vi "sortSTData.vi"(8 "error in (no error)":errorcluster, 9 "channelData":T1(array[cluster]), 10 "times":dbl[](array[numeric]), 11 "ScriptEventList in":refnum<class "ScriptEventList.lvclass">) -> (0 "error out":errorcluster, 2 "sortedData":T1(array[cluster]), 3 "ScriptEventList out":refnum<class "ScriptEventList.lvclass">)   [LabVIEW 2011, in "Tools.lvlib" / "Scripting.lvlib" / "ScriptEventList.lvclass"]
uses:
  ScriptEventList.lvclass
  DatabaseHelpers/Database Objects/Channel/Channel.lvclass
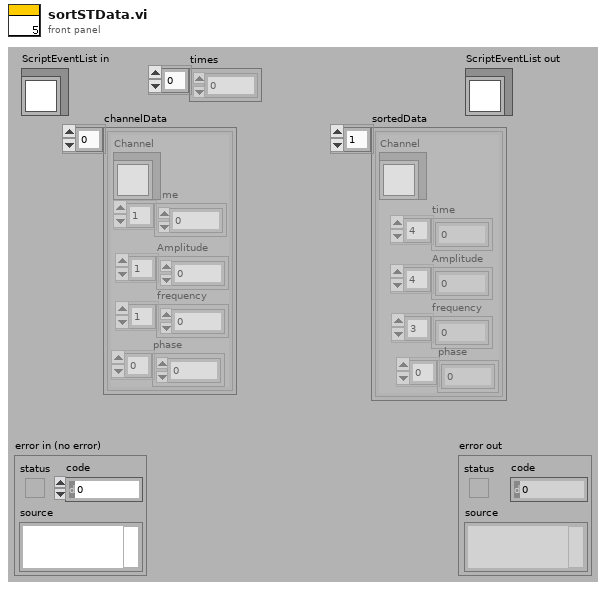
[diagram p1: front panel]
types:
  T1 = cluster{"Channel":refnum<class "Channel.lvclass">, "time":dbl[], "Amplitude":dbl[], "frequency":dbl[], "phase":dbl[]}[]
  T2 = cluster{"Channel":refnum<class "Channel.lvclass">, "time":dbl[], "Amplitude":dbl[], "frequency":dbl[], "phase":dbl[]}
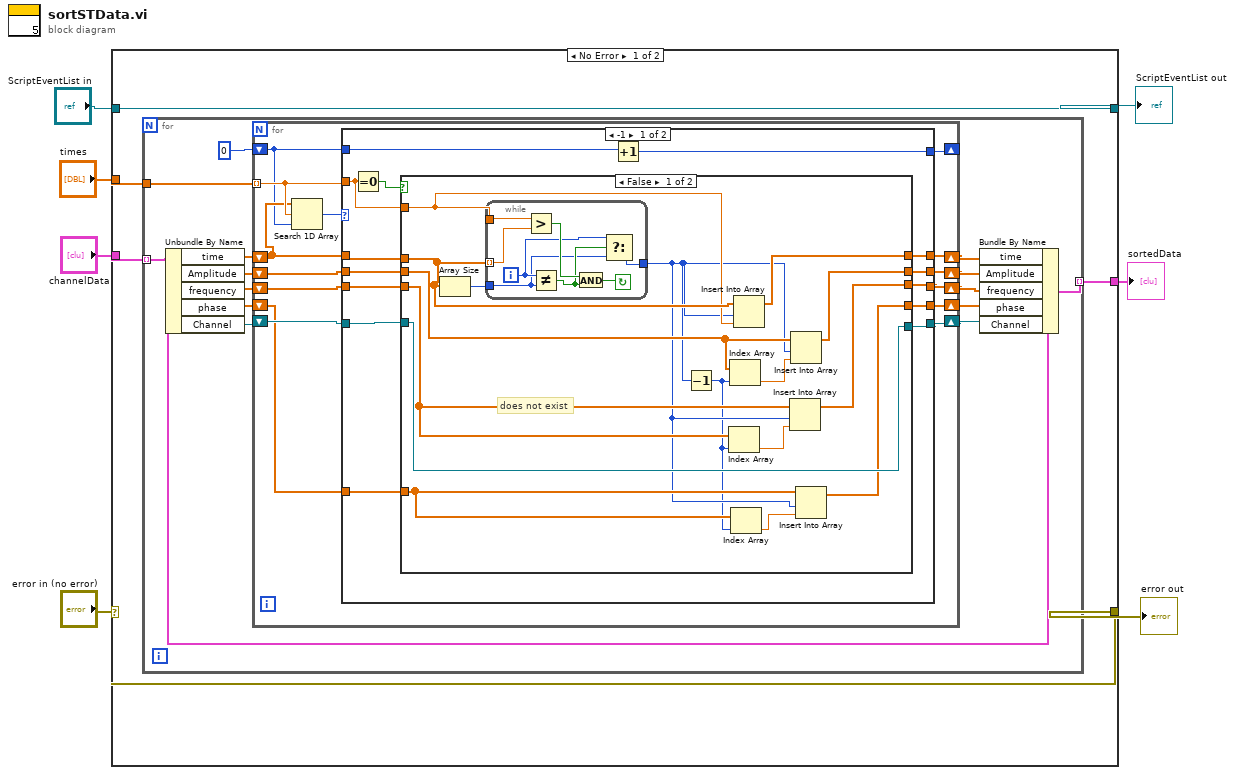
[diagram p0: block diagram]
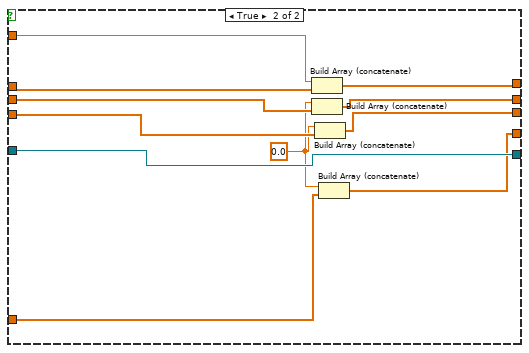
[diagram p2: hidden frame]
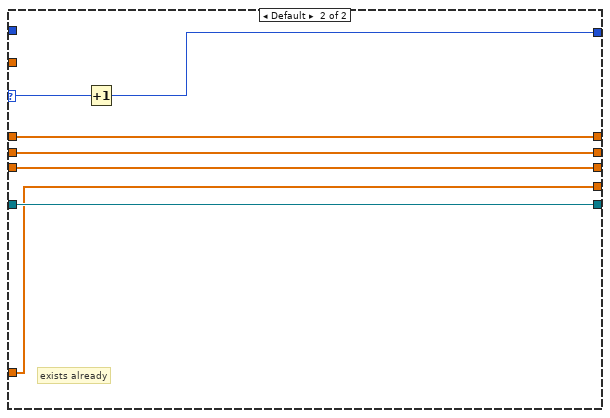
[diagram p3: hidden frame]
diagram:
  n1 = case shown="No Error" "error in (no error)" {
    selector: "error in (no error)" -> [w11 w98]
    tunnel: [w11 w98] -> w6
    tunnel: [w12 w97] -> w4
    tunnel: "ScriptEventList in" -> [w12 w97]
    tunnel: "times" -> [w9 _]
    tunnel: "channelData" -> [w10 _]
    tunnel: [w8 _] -> w1
    frame No Error {
      n2 = for {
        tunnel: w10 -> [w21] mode=indexing
        tunnel: w9 -> [w26]
        tunnel: [w17] -> w8 mode=indexing
        n3 = Unbundle By Name(w21) -> ("time"=w23:dbl[], "Amplitude"=w25:dbl[], "frequency"=w24:dbl[], "phase"=w15:dbl[], "Channel"=w16:refnum<class "Channel.lvclass">)
        n4 = for {
          tunnel: w26 -> [w32] mode=indexing
          shift-right: [w33] -> w20
          shift-left: w23 -> [w31]
          shift-right: [w34] -> w19
          shift-left: w25 -> [w39]
          shift-right: [w35] -> w18
          shift-left: w24 -> [w38]
          shift-right: [w36] -> w14
          shift-left: w16 -> [w37]
          shift-right: [w29] -> _
          shift-left: 0 -> [w30]
          shift-right: [w27] -> w13
          shift-left: w15 -> [w28]
          n5 = Search 1D Array(1D array=w31, element=w32, start index (0)=w30) -> (index of element=w40:i32)
          n6 = case shown="-1" w40 {
            selector: w40 -> [_ w92]
            tunnel: w31 -> [w52 w93]
            tunnel: w39 -> [w51 w94]
            tunnel: w38 -> [w50 w95]
            tunnel: w37 -> [w49 w96]
            tunnel: [w45 w96] -> w36
            tunnel: [w46 w95] -> w35
            tunnel: [w47 w94] -> w34
            tunnel: [w48 w93] -> w33
            tunnel: w32 -> [w53 _]
            tunnel: w30 -> [w44 _]
            tunnel: [w43 w91] -> w29
            tunnel: w28 -> [w42 w90]
            tunnel: [w41 w90] -> w27
            frame -1 {
              # "does not exist"
              n7 = Equal To 0?(x=w53) -> (x = 0?=w54:bool)
              n8 = case shown="False" w54 {
                tunnel: w53 -> [w69 w87]
                tunnel: w52 -> [w70 w89]
                tunnel: w51 -> [w67 w86]
                tunnel: w50 -> [w63 w84]
                tunnel: w49 -> [w61 w82]
                tunnel: [w68 w88] -> w48
                tunnel: [w65 w85] -> w47
                tunnel: [w62 w83] -> w46
                tunnel: [w61 w82] -> w45
                tunnel: w42 -> [w59 w81]
                tunnel: [w55 w79] -> w41
                frame False {
                  n9 = Array Size(array=w70) -> (size(s)=w60:i32)
                  n10 = while {
                    tunnel: w69 -> [w78]
                    tunnel: w70 -> [w77] mode=indexing
                    tunnel: [w73] -> w58
                    tunnel: w60 -> [w71]
                    i -> [w72]
                    stop <- w75 continue-if-true
                    n11 = Greater?(x=w78, y=w77) -> (0:w76:bool)
                    n12 = Not Equal?(x=w72, y=w71) -> (x != y?=w74:bool)
                    n13 = And(x=w76, y=w74) -> (x .and. y?=w75:bool)
                    n14 = Select(t=w72, s=w74, f=w71) -> (s? t:f=w73:i32)
                  }
                  n15 = Decrement(x=w58) -> (x-1=w57:i32)
                  n16 = Index Array(array=w63, index=w57) -> (element=w64:dbl)
                  n17 = Index Array(array=w67, index=w57) -> (element=w66:dbl)
                  n18 = Index Array(array=w59, index=w57) -> (element=w56:dbl)
                  n19 = Insert Into Array(array=w70, index=w58, new element=w69) -> (w68:dbl[])
                  n20 = Insert Into Array(array=w63, index=w58, new element=w64) -> (w62:dbl[])
                  n21 = Insert Into Array(array=w67, index=w58, new element=w66) -> (w65:dbl[])
                  n22 = Insert Into Array(array=w59, index=w58, new element=w56) -> (w55:dbl[])
                }
                frame True {
                  w80 = 0.0
                  n23 = Build Array (concatenate)(w87, w89) -> (w88:dbl[])
                  n24 = Build Array (concatenate)(w80, w86) -> (w85:dbl[])
                  n25 = Build Array (concatenate)(w80, w84) -> (w83:dbl[])
                  n26 = Build Array (concatenate)(w80, w81) -> (w79:dbl[])
                }
              }
              n27 = Increment(x=w44) -> (x+1=w43:i32)
            }
            frame Default {
              # "exists already"
              n28 = Increment(x=w92) -> (x+1=w91:i32)
            }
          }
        }
        n29 = Bundle By Name(cluster=w21, "time"=w20, "Amplitude"=w19, "frequency"=w18, "phase"=w13, "Channel"=w14) -> (w17:T2)
      }
    }
    frame Error {
    }
  }
  "error out" <- w6
  "ScriptEventList out" <- w4
  "sortedData" <- w1
